vi "数据查询_校准查询.vi"() -> ()   [LabVIEW 2016]
uses:
  <vilib>/Utility/miscctls.llb/LVRowAndColumnUnsignedTypeDef.ctl
  <vilib>/Utility/miscctls.llb/LVPointTypeDef.ctl
  <userlib>/_OpenG.lib/array/array.llb/Sort 2D Array (String)__ogtk.vi
panel:
  in  "显示行数":i32=100
  in  "下拉列表":string(xcontrol)
  in  "导出":bool
  in  "查询":bool
  in  "结束日期":string="2050/01/01"
  in  "起始日期":string="2010/01/01"
  out "数据表":string[][](table)
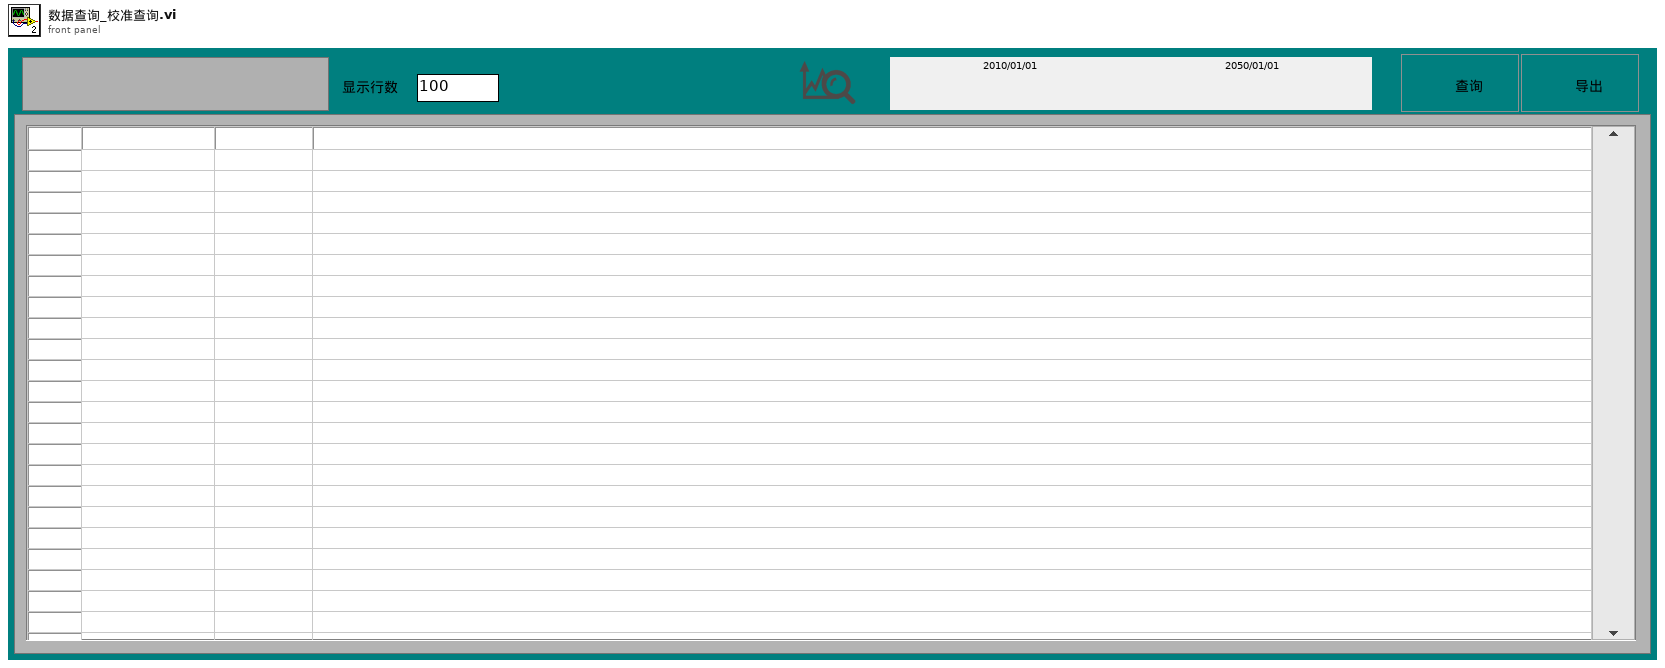
[diagram p1: front panel]
types:
  T1 = enum8{"Enabled", "Disabled", "Disabled and Grayed Out"}
  T2 = typedef "LVRowAndColumnUnsignedTypeDef.ctl" = cluster{"Row":u32, "Column":u32}
  T3 = typedef "LVPointTypeDef.ctl" = cluster{"Horizontal":i16, "Vertical":i16}
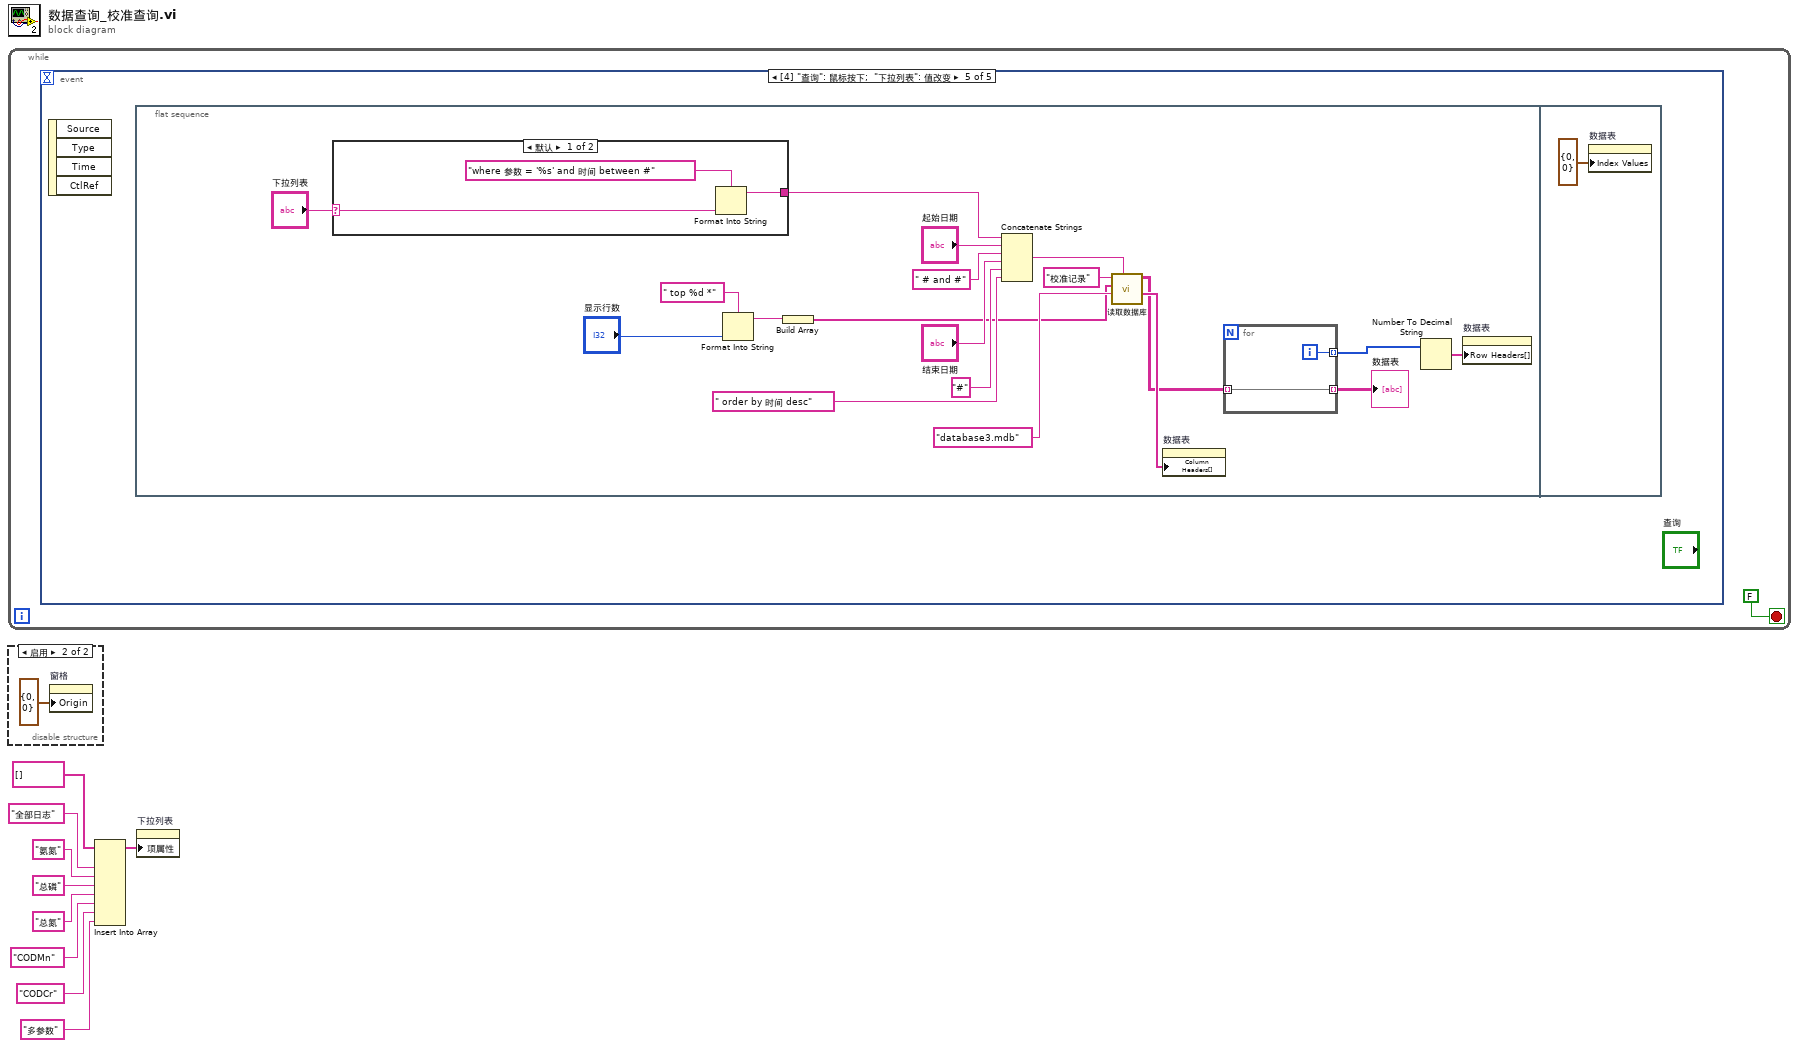
[diagram p0: block diagram]
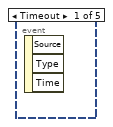
[diagram p2: hidden frame]
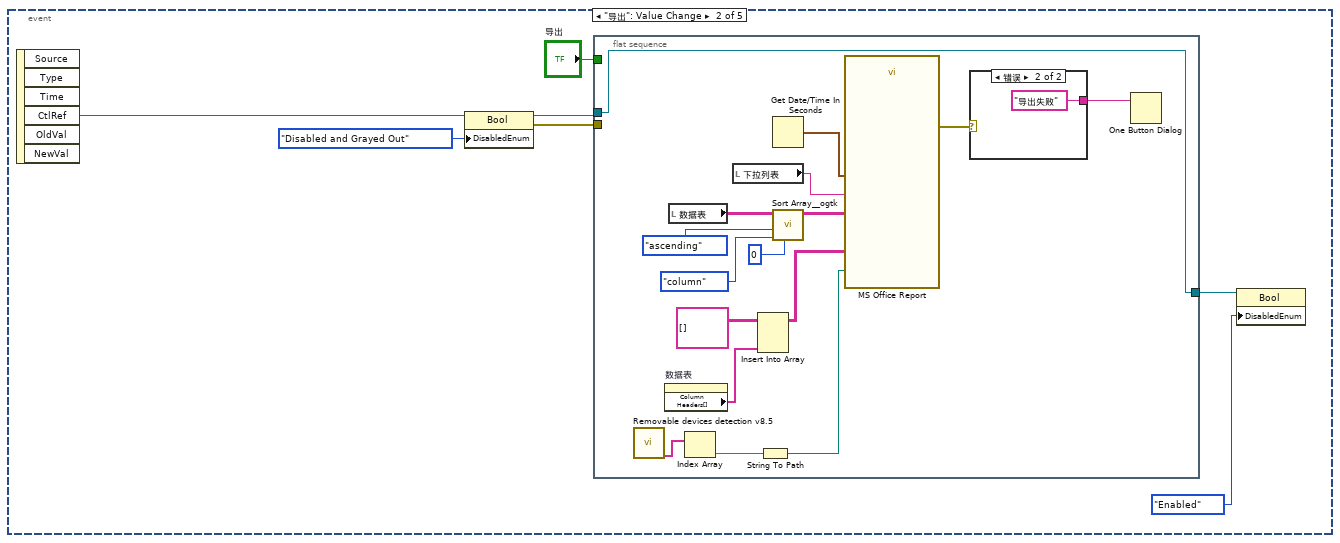
[diagram p3: hidden frame]
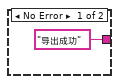
[diagram p4: hidden frame]
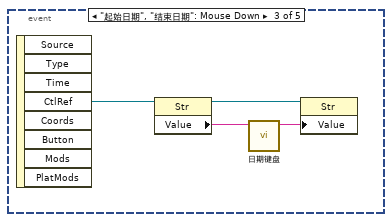
[diagram p5: hidden frame]
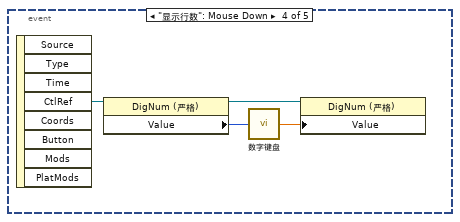
[diagram p6: hidden frame]
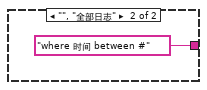
[diagram p7: hidden frame]
diagram:
  n1 = while {
    stop <- FALSE stop-if-true
    n2 = event shown="[4] \"查询\": 鼠标按下;  \"下拉列表\": 值改变" {
      selector: _ -> [_ _ _ _ _]
      dyn-events: _ -> [_ _ _ _ _]
      timeout: _ -> [_ _ _ _ _]
      event Timeout {
        n3 = event-data() -> ()  [unwired: 1 in, 3 out]
      }
      event "导出": Value Change {
        n4 = event-data() -> ("CtlRef"=w11:refnum<vi>)  [unwired: 1 in, 5 out]
        n5 = property class="Bool"(reference=w11, "DisabledEnum"=T1."Disabled and Grayed Out" ("禁用")) -> (reference out=w15:refnum<vi>, error out=w16:errorcluster)  [unwired: 1 in]
        n6 = flat-sequence {
          tunnel: w16 -> [_]
          tunnel: [w26] -> w14
          tunnel: w15 -> [w26]
          tunnel: "导出" -> [_]
          frame #0 {
            n7 = call "Removable devices detection v8.5.vi"() -> ("Removable"=w23:string[])  [unwired: 4 out]
            n8 = property on="数据表" class="Tbl (严格)"() -> ("Column Headers[]"=w19:string[])  [unwired: 2 in, 2 out]
            n9 = local read "数据表"() -> (w32:string[][])
            n10 = Index Array(array=w23) -> (element=w22:string)  [unwired: 1 in]
            n11 = local read "下拉列表"() -> (w27:string)
            n12 = Insert Into Array(array=string[][] [], new element=w19) -> (w18:string[][])  [unwired: 2 in]
            n13 = String To Path(string=w22) -> (path=w21:path)
            n14 = Get Date/Time In Seconds() -> (seconds since 1Jan1904=w33:timestamp)
            n15 = call-poly <userlib>:"Sort Array__ogtk.vi"("Column/Row to Sort By"=u32 0, "Sort By in"=enum16{"row", "column"}."column", "Order"=enum16{"ascending", "descending"}."ascending", "Array in"=w32) -> ("Sorted Array out"=w31:string[][])  [unwired: 4 in, 3 out]
            n16 = call "MS Office Report"("Path to Save Report"=w21, "导出日期"=w33, "监测参数"=w27, "数据输入"=w31, "字段定义"=w18) -> ("error out"=w25:errorcluster)  [unwired: 21 in, 1 out]
            n17 = case shown="错误" w25 {
              tunnel: ["导出成功" ("消息") "导出失败" ("消息")] -> w24
              frame No Error {
              }
              frame Error {
              }
            }
            n18 = One Button Dialog(message=w24) -> ()  [unwired: 1 in, 1 out]
          }
        }
        n19 = property class="Bool"(reference=w14, "DisabledEnum"=T1."Enabled" ("禁用")) -> ()  [unwired: 1 in, 2 out]
      }
      event "起始日期", "结束日期": Mouse Down {
        n20 = event-data() -> ("CtlRef"=w39:refnum<vi>)  [unwired: 1 in, 7 out]
        n21 = property class="Str"(reference=w39) -> (reference out=w37:refnum<vi>, "Value"=w38:string)  [unwired: 1 in, 1 out]
        n22 = call "日期键盘.vi"("原值"=w38) -> ("x+y"=w36:string)  [unwired: 10 in]
        n23 = property class="Str"(reference=w37, "Value"=w36) -> ()  [unwired: 1 in, 2 out]
      }
      event "显示行数": Mouse Down {
        n24 = event-data() -> ("CtlRef"=w43:refnum<vi>)  [unwired: 1 in, 7 out]
        n25 = property class="DigNum (严格)"(reference=w43) -> (reference out=w42:refnum<vi>, "Value"=w41:i32)  [unwired: 1 in, 1 out]
        n26 = call "数字键盘.vi"("OldNumber"=w41) -> ("NewNumber"=w40:sgl)
        n27 = property class="DigNum (严格)"(reference=w42, "Value"=w40) -> ()  [unwired: 1 in, 2 out]
      }
      event "查询": Mouse Down; "下拉列表": Value Change {
        n28 = event-data() -> ()  [unwired: 1 in, 4 out]
        n29 = flat-sequence {
          frame #0 {
            n30 = case shown="默认" "下拉列表" {
              selector: "下拉列表" -> [w63 _]
              tunnel: [w65 "where 时间 between #" ("condition")] -> w52
              frame Default {
                n31 = Format Into String(format string="where 参数 = '%s' and 时间 between #" ("condition"), w63) -> (resulting string=w65:string)  [unwired: 2 in, 1 out]
              }
              frame "", "全部日志" {
              }
            }
            n32 = Format Into String(format string=" top %d *" ("格式字符串"), "显示行数") -> (resulting string=w46:string)  [unwired: 2 in, 1 out]
            n33 = Build Array(w46) -> (w44:string[])
            n34 = Concatenate Strings(w52, "起始日期", " # and #" ("condition"), "结束日期", "#" ("condition"), " order by 时间 desc" ("字符串")) -> (w61:string)
            n35 = call "读取数据库.vi"("condition"=w61, "database"="database3.mdb", "显示项"=w44, "组合框"="校准记录" ("database")) -> ("columns"=w57:string[], "表格"=w49:string[][])  [unwired: 4 in, 2 out]
            n36 = property on="数据表" class="Tbl (严格)"("Column Headers[]"=w57) -> ()  [unwired: 2 in, 2 out]
            n37 = for {
              tunnel: w49 -> [w67] mode=indexing
              tunnel: [w68] -> w55 mode=indexing
              tunnel: [w67] -> w50 mode=indexing
              i -> [w68]
            }
            "数据表" <- w50
            n38 = Number To Decimal String(number=w55) -> (decimal integer string=w54:string[])  [unwired: 1 in]
            n39 = property on="数据表" class="Tbl (严格)"("Row Headers[]"=w54) -> ()  [unwired: 2 in, 2 out]
          }
          frame #1 {
            n40 = property on="数据表" class="Tbl (严格)"("Index Values"=T2 {"Row"=0, "Column"=0} ("索引值")) -> ()  [unwired: 2 in, 2 out]
          }
        }
      }
    }
  }
  n41 = disable-structure shown="启用" {
    frame Disabled {
    }
    frame Enabled {
      n42 = property on="窗格" class="Pane"("Origin"=T3 {"Horizontal"=0, "Vertical"=0} ("原点")) -> ()  [unwired: 2 in, 2 out]
    }
  }
  n43 = Insert Into Array(array=string[] [], new element #1="全部日志" ("新元素/子数组"), new element #2="氨氮" ("新元素/子数组"), new element #3="总磷" ("新元素/子数组"), new element #4="总氮" ("新元素/子数组"), new element #5="CODMn" ("新元素/子数组"), new element #6="CODCr" ("新元素/子数组"), new element #7="多参数" ("新元素/子数组")) -> (w1:string[])  [unwired: 1 in]
  n44 = property on="下拉列表" class="下拉列表 (严格)"("项属性"=w1) -> ()  [unwired: 2 in, 2 out]
